vi "S2C_UNITHERM_Poly_TestBed.vi"() -> ()   [LabVIEW 2015]
uses:
  S2C_UNITHERM_Poly_Initialize.vi
  S2C_UNITHERM_Poly_Reset.vi
  S2C_UNITHERM_Poly_Identify.vi
  S2C_UNITHERM_Poly_ProtectOn.vi
  S2C_UNITHERM_Poly_ProtectOff.vi
  S2C_UNITHERM_Poly_SelfTest.vi
  S2C_UNITHERM_Poly_CustCmd.vi
  S2C_UNITHERM_Poly_LoadSet.vi
  S2C_UNITHERM_Poly_LoadClear.vi
  S2C_UNITHERM_Poly_Status.vi
  S2C_UNITHERM_Poly_CrestFactor.vi
  S2C_UNITHERM_Poly_RmsCurrent.vi
  S2C_UNITHERM_Poly_PeakCurrent.vi
  S2C_UNITHERM_Poly_RmsVoltage.vi
  S2C_UNITHERM_Poly_PeakVoltage.vi
panel:
  out "Error Out":errorcluster
  in  "Error In":errorcluster
  out "Response":T1
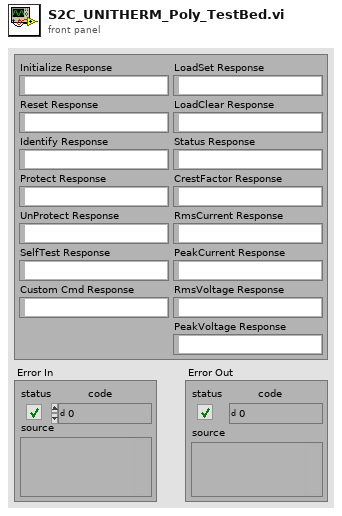
[diagram p1: front panel]
types:
  T1 = cluster{"Initialize Response":string, "Reset Response":string, "Identify Response":string, "Protect Response":string, "UnProtect Response":string, "SelfTest Response":string, "Custom Cmd Response":string, "LoadSet Response":string, "LoadClear Response":string, "Status Response":string, "CrestFactor Response":string, "RmsCurrent Response":string, "PeakCurrent Response":string, "RmsVoltage Response":string, "PeakVoltage Response":string}
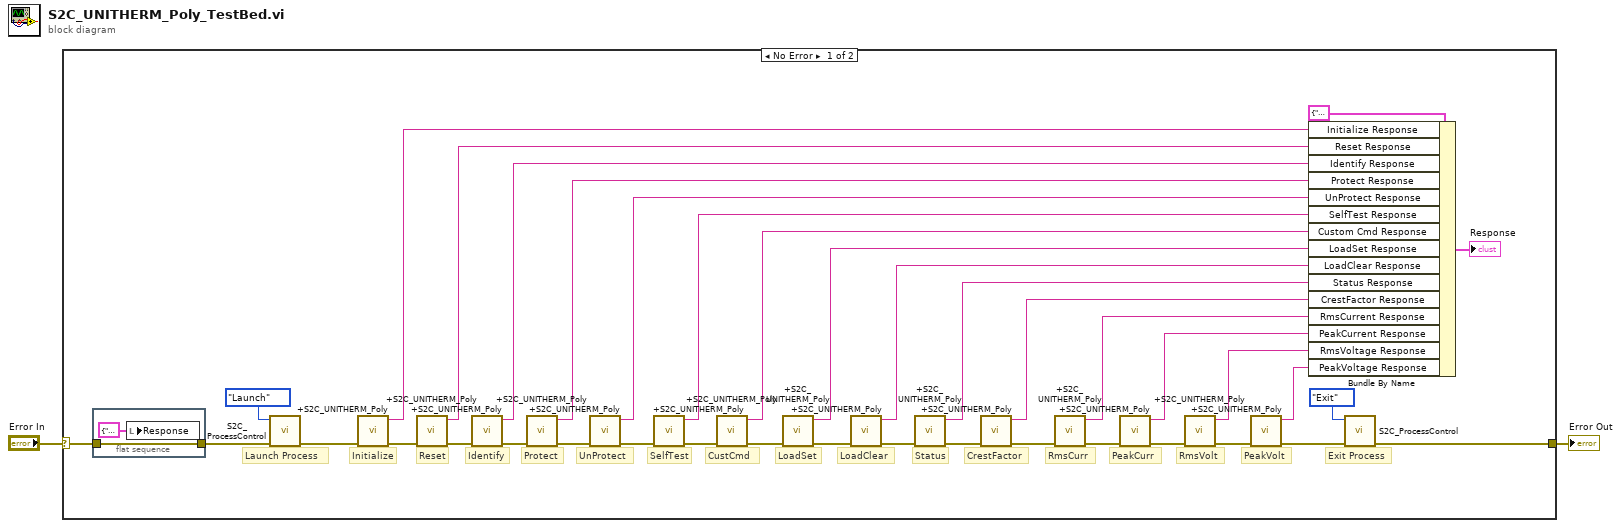
[diagram p0: block diagram]
diagram:
  n1 = case shown="No Error" "Error In" {
    selector: "Error In" -> [w17 w43]
    tunnel: [w36 w43] -> w1
    frame No Error {
      # "PeakVolt"
      # "RmsVolt"
      # "PeakCurr"
      # "RmsCurr"
      # "CrestFactor"
      # "Status"
      # "LoadClear"
      # "SelfTest"
      # "UnProtect"
      # "Protect"
      # "Identify"
      # "Reset"
      # "CustCmd"
      # "LoadSet"
      # "Exit Process"
      # "Initialize"
      # "Launch Process"
      n2 = flat-sequence {
        tunnel: w17 -> [w41]
        tunnel: [w41] -> w16
        frame #0 {
          n3 = local write "Response"(T1 {"Initialize Response"="", "Reset Response"="", "Identify Response"="", "Protect Response"="", "UnProtect Response"="", "SelfTest Response"="", "Custom Cmd Response"="", "LoadSet Response"="", "LoadClear Response"="", "Status Response"="", "CrestFactor Response"="", "RmsCurrent Response"="", "PeakCurrent Response"="", "RmsVoltage Response"="", "PeakVoltage Response"=""} ("Response")) -> ()
        }
      }
      n4 = call "S2C_ProcessControl.vi"("Error In"=w16, "Action"=enum16{"Launch", "Exit"}."Launch") -> ("Error Out"=w39:errorcluster)  [unwired: 9 in]
      n5 = call-poly "+S2C_UNITHERM_Poly.vi"("Error In"=w39) -> ("Error Out"=w38:errorcluster, "Response"=w18:string)  [unwired: 9 in]
      n6 = call-poly "+S2C_UNITHERM_Poly.vi"("Error In"=w38) -> ("Error Out"=w12:errorcluster, "Response"=w19:string)  [unwired: 9 in]
      n7 = call-poly "+S2C_UNITHERM_Poly.vi"("Error In"=w12) -> ("Error Out"=w11:errorcluster, "Response"=w20:string)  [unwired: 9 in]
      n8 = call-poly "+S2C_UNITHERM_Poly.vi"("Error In"=w11) -> ("Error Out"=w9:errorcluster, "Response"=w21:string)  [unwired: 9 in]
      n9 = call-poly "+S2C_UNITHERM_Poly.vi"("Error In"=w9) -> ("Error Out"=w10:errorcluster, "Response"=w22:string)  [unwired: 9 in]
      n10 = call-poly "+S2C_UNITHERM_Poly.vi"("Error In"=w10) -> ("Error Out"=w13:errorcluster, "Response"=w23:string)  [unwired: 9 in]
      n11 = call-poly "+S2C_UNITHERM_Poly.vi"("Error In"=w13) -> ("Error Out"=w15:errorcluster, "Response"=w24:string)  [unwired: 9 in]
      n12 = call-poly "+S2C_UNITHERM_Poly.vi"("Error In"=w15) -> ("Error Out"=w14:errorcluster, "Response"=w25:string)  [unwired: 9 in]
      n13 = call-poly "+S2C_UNITHERM_Poly.vi"("Error In"=w14) -> ("Error Out"=w8:errorcluster, "Response"=w26:string)  [unwired: 9 in]
      n14 = call-poly "+S2C_UNITHERM_Poly.vi"("Error In"=w8) -> ("Error Out"=w7:errorcluster, "Response"=w27:string)  [unwired: 9 in]
      n15 = call-poly "+S2C_UNITHERM_Poly.vi"("Error In"=w7) -> ("Error Out"=w6:errorcluster, "Response"=w28:string)  [unwired: 9 in]
      n16 = call-poly "+S2C_UNITHERM_Poly.vi"("Error In"=w6) -> ("Error Out"=w3:errorcluster, "Response"=w29:string)  [unwired: 9 in]
      n17 = call-poly "+S2C_UNITHERM_Poly.vi"("Error In"=w3) -> ("Error Out"=w4:errorcluster, "Response"=w30:string)  [unwired: 9 in]
      n18 = call-poly "+S2C_UNITHERM_Poly.vi"("Error In"=w4) -> ("Error Out"=w5:errorcluster, "Response"=w31:string)  [unwired: 9 in]
      n19 = call-poly "+S2C_UNITHERM_Poly.vi"("Error In"=w5) -> ("Error Out"=w35:errorcluster, "Response"=w32:string)  [unwired: 9 in]
      n20 = Bundle By Name(cluster=T1 {"Initialize Response"="", "Reset Response"="", "Identify Response"="", "Protect Response"="", "UnProtect Response"="", "SelfTest Response"="", "Custom Cmd Response"="", "LoadSet Response"="", "LoadClear Response"="", "Status Response"="", "CrestFactor Response"="", "RmsCurrent Response"="", "PeakCurrent Response"="", "RmsVoltage Response"="", "PeakVoltage Response"=""} ("Cluster"), "Initialize Response"=w18, "Reset Response"=w19, "Identify Response"=w20, "Protect Response"=w21, "UnProtect Response"=w22, "SelfTest Response"=w23, "Custom Cmd Response"=w24, "LoadSet Response"=w25, "LoadClear Response"=w26, "Status Response"=w27, "CrestFactor Response"=w28, "RmsCurrent Response"=w29, "PeakCurrent Response"=w30, "RmsVoltage Response"=w31, "PeakVoltage Response"=w32) -> (→"Response":T1)
      n21 = call "S2C_ProcessControl.vi"("Error In"=w35, "Action"=enum16{"Launch", "Exit"}."Exit") -> ("Error Out"=w36:errorcluster)  [unwired: 9 in]
    }
    frame Error {
    }
  }
  "Error Out" <- w1
